vi "File.Write to CSV.vi"(0 "Folder":path, 1 "FileRootName":string, 2 "Header":string[](array[string]), 5 "1D":string[](array[string]), 7 "2D":string[][](array[string]), 9 "Add Quotes":bool, 11 "error in":errorcluster, 12 "Append Time to Filename":bool, 13 "Append Date to Filename":bool) -> (4 "File Path":path, 15 "error out":errorcluster)   [LabVIEW 2024, in "EQMF.lvlib" / "File Utils.lvlib"]
uses:
  File Utils.lvlib
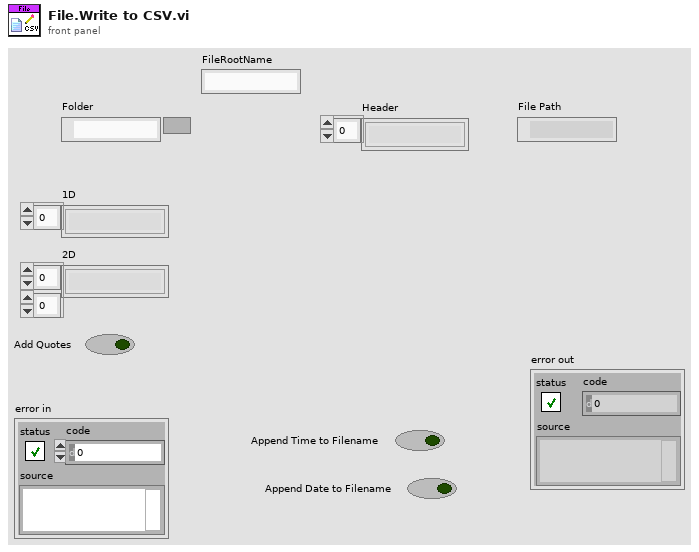
[diagram p1: front panel]
types:
  T1 = enum16{"open", "replace", "create", "open or create", "replace or create", "replace or create with confirmation"}
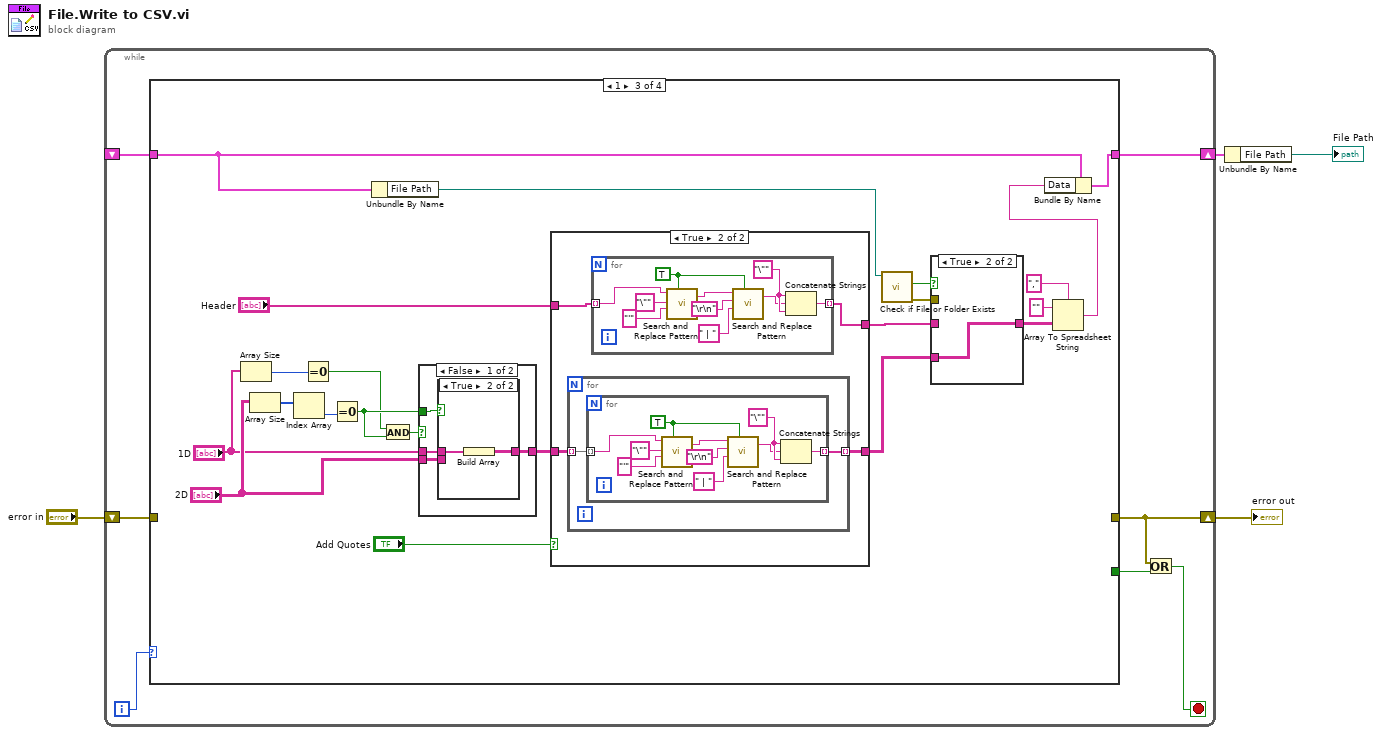
[diagram p0: block diagram]
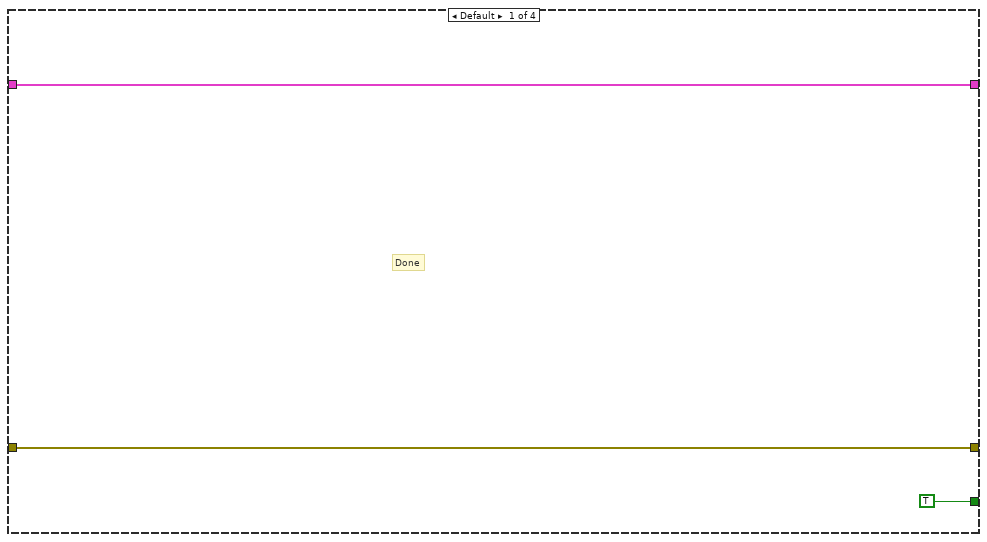
[diagram p2: hidden frame]
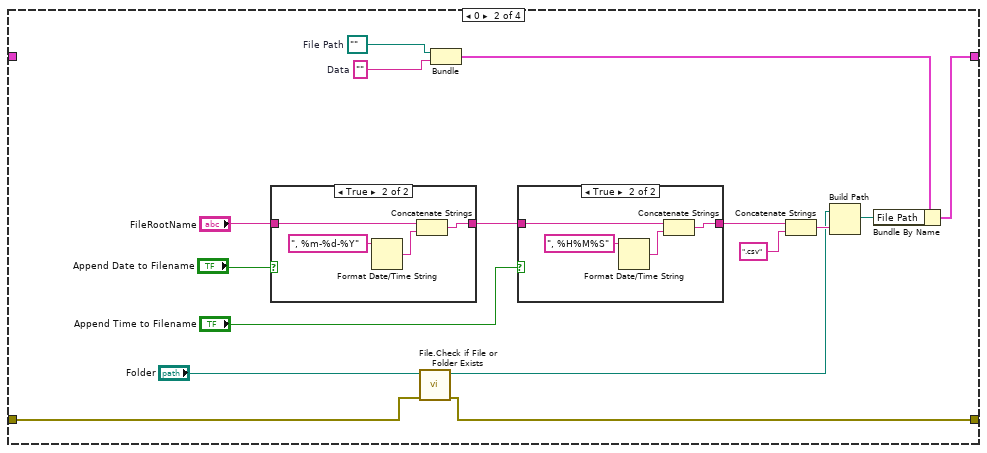
[diagram p3: hidden frame]
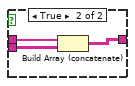
[diagram p7: hidden frame]
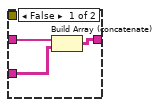
[diagram p8: hidden frame]
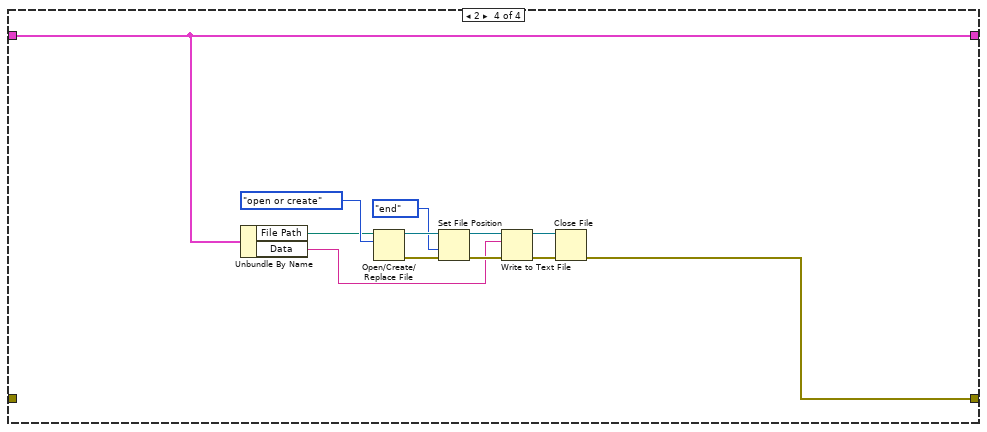
[diagram p10: hidden frame]
diagram:
  n1 = while {
    shift-right: [w8] -> w3
    shift-left: "error in" -> [w10]
    shift-right: [w6] -> w2
    shift-left: _ -> [w5]
    i -> [w11]
    stop <- w9 stop-if-true
    n2 = case shown="1" w11 {
      tunnel: w10 -> [w12 w17 _ _]
      tunnel: [w12 w21 _ w108] -> w8
      tunnel: [TRUE _ _ _] -> w7
      tunnel: [w13 w15 w61 w105] -> w6
      tunnel: w5 -> [w13 _ w62 w105]
      frame Default {
        # "Done"
      }
      frame 0 {
        w20 = path ""  # File Path
        w19 = ""  # Data
        n3 = case shown="True" "Append Date to Filename" {
          tunnel: "FileRootName" -> [w36 w40]
          tunnel: [w36 w37] -> w27
          frame False {
          }
          frame True {
            n4 = Format Date/Time String(time format string (%c)=", %m-%d-%Y") -> (date/time string=w38:string)  [unwired: 2 in]
            n5 = Concatenate Strings(w40, w38) -> (w37:string)
          }
        }
        n6 = call "File.Check if File or Folder Exists.vi"("error in"=w17, "Path"="Folder") -> ("error out"=w21:errorcluster, "Dup Path"=w22:path)  [unwired: 5 in, 3 out]
        n7 = Bundle("File Path"=w20, "Data"=w19) -> (w16:cluster{"File Path":path, "Data":string})  [unwired: 1 in]
        n8 = case shown="True" "Append Time to Filename" {
          tunnel: w27 -> [w31 w35]
          tunnel: [w31 w32] -> w29
          frame False {
          }
          frame True {
            n9 = Format Date/Time String(time format string (%c)=", %H%M%S") -> (date/time string=w33:string)  [unwired: 2 in]
            n10 = Concatenate Strings(w35, w33) -> (w32:string)
          }
        }
        n11 = Concatenate Strings(w29, ".csv" ("string")) -> (w24:string)
        n12 = Build Path(base path=w22, name or relative path=w24) -> (appended path=w18:path)
        n13 = Bundle By Name(cluster=w16, "File Path"=w18) -> (w15:cluster{"File Path":path, "Data":string})
      }
      frame 1 {
        n14 = Array Size(array="1D") -> (size(s)=w57:i32)
        n15 = Array Size(array="2D") -> (size(s)=w55:i32[])
        n16 = Index Array(array=w55) -> (element=w56:i32)  [unwired: 1 in]
        n17 = Equal To 0?(x=w57) -> (x = 0?=w58:bool)
        n18 = Equal To 0?(x=w56) -> (x = 0?=w60:bool)
        n19 = Unbundle By Name(w62) -> ("File Path"=w45:path)
        n20 = And(x=w58, y=w60) -> (x .and. y?=w59:bool)
        n21 = case shown="False" w59 {
          tunnel: [w66 w70] -> w47
          tunnel: "1D" -> [w65 w72]
          tunnel: "2D" -> [w64 w71]
          tunnel: w60 -> [w63 _]
          frame False {
            n22 = case shown="True" w63 {
              tunnel: [w67 w68] -> w66
              tunnel: w65 -> [_ w69]
              tunnel: w64 -> [w67 _]
              frame False {
              }
              frame True {
                n23 = Build Array(w69) -> (w68:string[][])
              }
            }
          }
          frame True {
            n24 = Build Array (concatenate)(w72, w71) -> (w70:string[][])
          }
        }
        n25 = case shown="True" "Add Quotes" {
          tunnel: w47 -> [w78 w82]
          tunnel: [w78 w81] -> w49
          tunnel: [w77 w80] -> w42
          tunnel: "Header" -> [w77 w79]
          frame False {
          }
          frame True {
            n26 = for {
              tunnel: w82 -> [w94] mode=indexing
              tunnel: [w93] -> w81 mode=indexing
              n27 = for {
                tunnel: w94 -> [w100] mode=indexing
                tunnel: [w103] -> w93 mode=indexing
                w98 = TRUE ("replace all? (F)")
                w104 = "\""
                n28 = call <vilib>:"Search and Replace Pattern.vi"("string"=w100, "regular expression (\"\")"="\"", "replace string (\"\")"="'", "replace all? (F)"=w98) -> ("result string"=w99:string)  [unwired: 1 in, 1 out]
                n29 = call <vilib>:"Search and Replace Pattern.vi"("string"=w99, "regular expression (\"\")"="\r\n", "replace string (\"\")"=" | ", "replace all? (F)"=w98) -> ("result string"=w97:string)  [unwired: 1 in, 1 out]
                n30 = Concatenate Strings(w104, w97, w104) -> (w103:string)
              }
            }
            n31 = for {
              tunnel: w79 -> [w88] mode=indexing
              tunnel: [w91] -> w80 mode=indexing
              w86 = TRUE ("replace all? (F)")
              w92 = "\""
              n32 = call <vilib>:"Search and Replace Pattern.vi"("string"=w88, "regular expression (\"\")"="\"", "replace string (\"\")"="'", "replace all? (F)"=w86) -> ("result string"=w87:string)  [unwired: 1 in, 1 out]
              n33 = call <vilib>:"Search and Replace Pattern.vi"("string"=w87, "regular expression (\"\")"="\r\n", "replace string (\"\")"=" | ", "replace all? (F)"=w86) -> ("result string"=w85:string)  [unwired: 1 in, 1 out]
              n34 = Concatenate Strings(w92, w85, w92) -> (w91:string)
            }
          }
        }
        n35 = call <vilib>:"Check if File or Folder Exists.vi"("path"=w45) -> ("error out"=w44:errorcluster, "file or folder exists?"=w48:bool)  [unwired: 8 in, 1 out]
        n36 = case shown="True" w48 {
          tunnel: [w75 w76] -> w50
          tunnel: w42 -> [w74 _]
          tunnel: w49 -> [w73 w76]
          tunnel: w44 -> [_ _]
          frame False {
            n37 = Build Array (concatenate)(w74, w73) -> (w75:string[][])
          }
          frame True {
          }
        }
        n38 = Array To Spreadsheet String(delimiter (Tab)=",", array=w50, 3:"" ("format string")) -> (spreadsheet string=w43:string)
        n39 = Bundle By Name(cluster=w62, "Data"=w43) -> (w61:cluster{"File Path":path, "Data":string})
      }
      frame 2 {
        n40 = Unbundle By Name(w105) -> ("File Path"=w107:path, "Data"=w106:string)
        n41 = Open/Create/Replace File(file path (use dialog)=w107, operation (0:open)=T1."open or create") -> (refnum out=w112:refnum<file>, error out=w111:errorcluster)  [unwired: 4 in, 1 out]
        n42 = Set File Position(refnum=w112, from (0:start)=enum16{"start", "end", "current"}."end", error in=w111) -> (refnum out=w114:refnum<file>, error out=w109:errorcluster)  [unwired: 1 in]
        n43 = Write to Text File(file (use dialog)=w114, text=w106, error in=w109) -> (refnum out=w115:refnum<file>, error out=w116:errorcluster)  [unwired: 1 in, 1 out]
        n44 = Close File(refnum=w115, error in=w116) -> (error out=w108:errorcluster)  [unwired: 1 out]
      }
    }
    n45 = Or(x=w8, y=w7) -> (x .or. y?=w9:bool)
  }
  "error out" <- w3
  n46 = Unbundle By Name(w2) -> ("File Path"=→"File Path":path)
